vi "MecaOdometry_Execute.vi"(6 "Initial Pose":T1={"TRANSLATION"={"X"=0.0, "Y"=0.0}, "ROTATION"={"VALUE"=0.0, "COS"=1.0, "SIN"=0.0}} {"ROTATION"."SIN" format="%13.4f"; "ROTATION"."COS" format="%13.4f"; "ROTATION"."VALUE" format="%13.4f"; "TRANSLATION"."Y" format="%14.3f"; "TRANSLATION"."X" format="%14.3f"}, 8 "Init":bool, 9 "Rotation":T3={"VALUE"=0.0, "COS"=1.0, "SIN"=0.0} {"SIN" format="%13.4f"; "COS" format="%13.4f"; "VALUE" format="%13.4f"}, 10 "Meca Module Positions":T4 {"RearRight" format="%19.3f"; "RearLeft" format="%19.3f"; "FrontRight" format="%19.3f"; "FrontLeft" format="%19.3f"}, 11 "MECA_DRIVE_KINEMATICS":T5={"FrontLeft"={"X"=0.0, "Y"=0.0}, "FrontRight"={"X"=0.0, "Y"=0.0}, "RearLeft"={"X"=0.0, "Y"=0.0}, "RearRight"={"X"=0.0, "Y"=0.0}, "InverseKinematics"=[[0.0, 1.0, -1.0, 0.0], [0.0, 1.0, 1.0, 0.0], [0.0, 1.0, 1.0, 0.0], [0.0, 1.0, -1.0, 0.0]], "ForwardKinematics"=[[0.0, 1.0, -1.0, 0.0], [0.0, 1.0, 1.0, 0.0], [0.0, 1.0, 1.0, 0.0], [0.0, 1.0, -1.0, 0.0]], "PrevCoR"={"X"=0.0, "Y"=0.0}} {"PrevCoR"."Y" format="%14.3f"; "PrevCoR"."X" format="%14.3f"; "RearRight"."Y" format="%14.3f"; "RearRight"."X" format="%14.3f"; "RearLeft"."Y" format="%14.3f"; "RearLeft"."X" format="%14.3f"; "FrontRight"."Y" format="%14.3f"; "FrontRight"."X" format="%14.3f"; "FrontLeft"."Y" format="%14.3f"; "FrontLeft"."X" format="%14.3f"}) -> (3 "Current Pose":T1={"TRANSLATION"={"X"=0.0, "Y"=0.0}, "ROTATION"={"VALUE"=0.0, "COS"=1.0, "SIN"=0.0}} {"ROTATION"."SIN" format="%13.4f"; "ROTATION"."COS" format="%13.4f"; "ROTATION"."VALUE" format="%13.4f"; "TRANSLATION"."Y" format="%14.3f"; "TRANSLATION"."X" format="%14.3f"}, 4 "MECA_DRIVE_ODOMETRY":T7={"POSE"={"TRANSLATION"={"X"=0.0, "Y"=0.0}, "ROTATION"={"VALUE"=0.0, "COS"=1.0, "SIN"=0.0}}, "GyroOffset"={"VALUE"=0.0, "COS"=1.0, "SIN"=0.0}, "PreviousAngle"={"VALUE"=0.0, "COS"=1.0, "SIN"=0.0}, "Kinematics"={"FrontLeft"={"X"=0.0, "Y"=0.0}, "FrontRight"={"X"=0.0, "Y"=0.0}, "RearLeft"={"X"=0.0, "Y"=0.0}, "RearRight"={"X"=0.0, "Y"=0.0}, "InverseKinematics"=[[0.0, 1.0, -1.0, 0.0], [0.0, 1.0, 1.0, 0.0], [0.0, 1.0, 1.0, 0.0], [0.0, 1.0, -1.0, 0.0]], "ForwardKinematics"=[[0.0, 1.0, -1.0, 0.0], [0.0, 1.0, 1.0, 0.0], [0.0, 1.0, 1.0, 0.0], [0.0, 1.0, -1.0, 0.0]], "PrevCoR"={"X"=0.0, "Y"=0.0}}, "PreviousWheelPositions"={"FrontLeft"=0.0, "FrontRight"=0.0, "RearLeft"=0.0, "RearRight"=0.0, "P"=FALSE}} {"PreviousWheelPositions"."RearRight" format="%19.3f"; "PreviousWheelPositions"."RearLeft" format="%19.3f"; "PreviousWheelPositions"."FrontRight" format="%19.3f"; "PreviousWheelPositions"."FrontLeft" format="%19.3f"; "Kinematics"."PrevCoR"."Y" format="%14.3f"; "Kinematics"."PrevCoR"."X" format="%14.3f"; "Kinematics"."RearRight"."Y" format="%14.3f"; "Kinematics"."RearRight"."X" format="%14.3f"; "Kinematics"."RearLeft"."Y" format="%14.3f"; "Kinematics"."RearLeft"."X" format="%14.3f"; "Kinematics"."FrontRight"."Y" format="%14.3f"; "Kinematics"."FrontRight"."X" format="%14.3f"; "Kinematics"."FrontLeft"."Y" format="%14.3f"; "Kinematics"."FrontLeft"."X" format="%14.3f"; "PreviousAngle"."SIN" format="%13.4f"; "PreviousAngle"."COS" format="%13.4f"; "PreviousAngle"."VALUE" format="%13.4f"; "GyroOffset"."SIN" format="%13.4f"; "GyroOffset"."COS" format="%13.4f"; "GyroOffset"."VALUE" format="%13.4f"; "POSE"."ROTATION"."SIN" format="%13.4f"; "POSE"."ROTATION"."COS" format="%13.4f"; "POSE"."ROTATION"."VALUE" format="%13.4f"; "POSE"."TRANSLATION"."Y" format="%14.3f"; "POSE"."TRANSLATION"."X" format="%14.3f"})   [LabVIEW 2019, in "Trajectory_Library.lvlib"]
doc: "SIngle call LabVIEW function to execute Mecanum Drive Odometry to calculate a relative or absolute POSE.\n \nInputs:\n - Mecanum_Drive_Kinematics -- cluster -- mecanum drive kinematics\n - Mecanum Wheel Positions -- array of cluster -- current wheel positions (distances).\n - Gyro Value -- rotation2d -- current gyro reading.\n - Init -- boolean -- Reset position to the value of Initial Pose. Odometry is calculated from this position.\n - Initial Pose -- Pose2d -- Pose to use when Init is TRUE. (Optional. Default: 0,0,0 )\n\nReturns\n - Current Pose -- Pose2d -- Current position calculated by Mecanum Odometry\n - Mecanum_Drive_Odometry -- cluster -- current value of the mecanum drive odometry cluster."
uses:
  TypeDef/POSE2D.ctl
  TypeDef/TRANSLATION2D.ctl
  TypeDef/ROTATION2D.ctl
  <vilib>/Analysis/Matrix/Datatypes/RealMatrix.ctl
  Pose2d_getRotation.vi
  Rotation2d_Minus.vi
  Rotation2d_UnaryMinus.vi
  Rotation2d_RotateBy.vi
  Rotation2d_CreateAngle.vi
  Rotation2d_CreateXY.vi
  Util_CalcDist.vi
  Trajectory_Library.lvlib
  <vilib>/Analysis/Matrix/NI_Matrix.lvlib
  TypeDef/MECA_DRIVE_KINEMATICS.ctl
  TypeDef/MECA_WHEEL_POSITIONS.ctl
  TypeDef/MECA_DRIVE_ODOMETRY.ctl
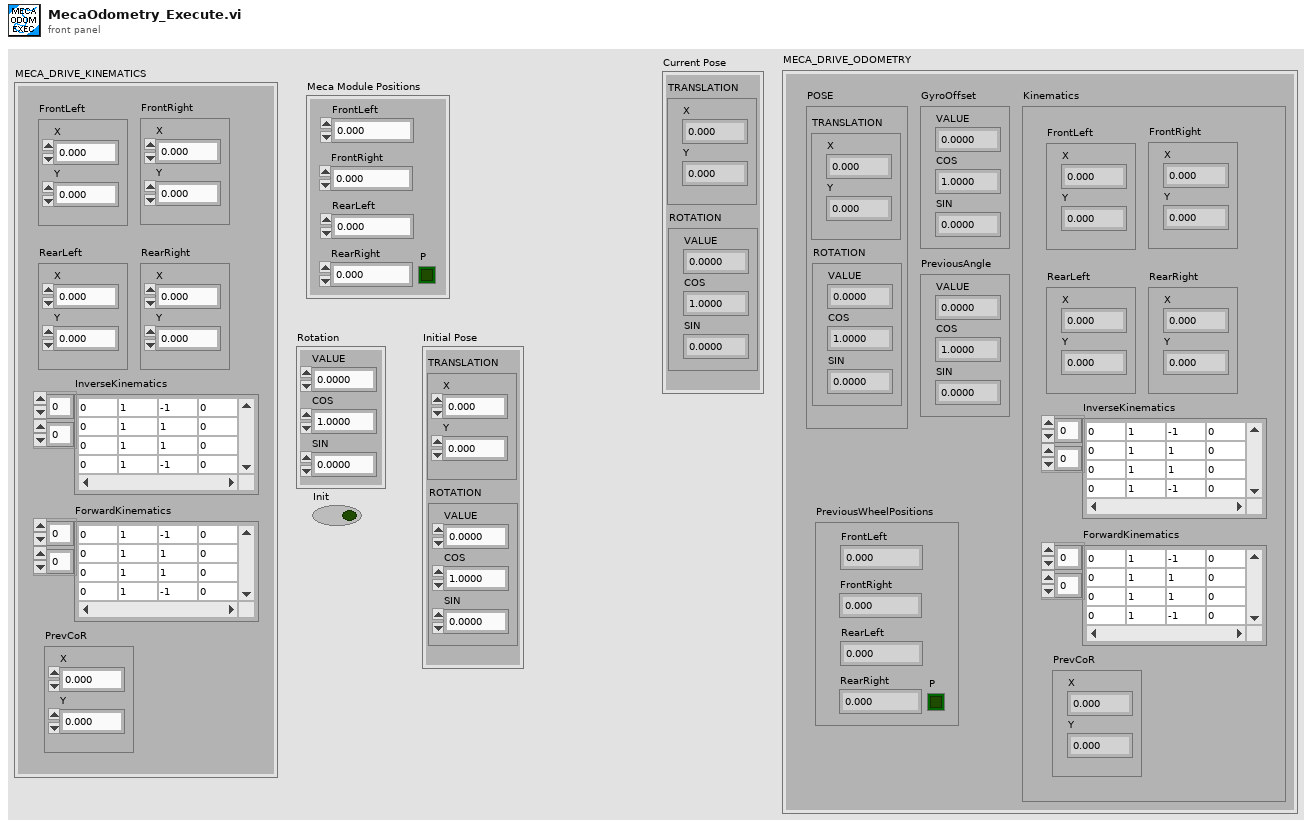
[diagram p1: front panel]
types:
  T1 = typedef "Trajectory_Library.lvlib/POSE2D.ctl" = cluster{"TRANSLATION":T2, "ROTATION":T3}
  T2 = typedef "Trajectory_Library.lvlib/TRANSLATION2D.ctl" = cluster{"X":dbl, "Y":dbl}
  T3 = typedef "Trajectory_Library.lvlib/ROTATION2D.ctl" = cluster{"VALUE":dbl, "COS":dbl, "SIN":dbl}
  T4 = typedef "Trajectory_Library.lvlib/MECA_WHEEL_POSITIONS.ctl" = cluster{"FrontLeft":dbl, "FrontRight":dbl, "RearLeft":dbl, "RearRight":dbl, "P":bool}
  T5 = typedef "Trajectory_Library.lvlib/MECA_DRIVE_KINEMATICS.ctl" = cluster{"FrontLeft":T2, "FrontRight":T2, "RearLeft":T2, "RearRight":T2, "InverseKinematics":T6, "ForwardKinematics":T6, "PrevCoR":T2}
  T6 = typedef "NI_Matrix.lvlib/RealMatrix.ctl" = dbl[][]
  T7 = typedef "Trajectory_Library.lvlib/MECA_DRIVE_ODOMETRY.ctl" = cluster{"POSE":T1, "GyroOffset":T3, "PreviousAngle":T3, "Kinematics":T5, "PreviousWheelPositions":T4}
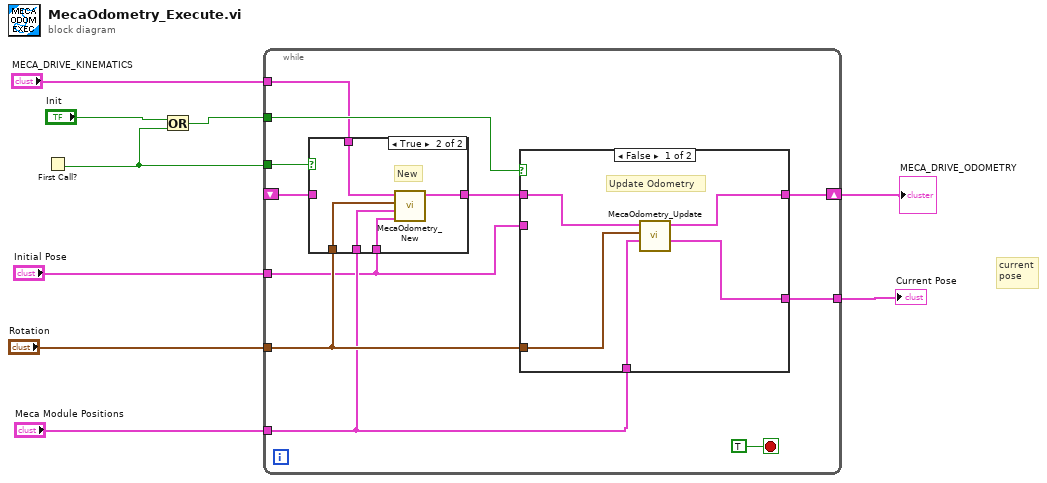
[diagram p0: block diagram]
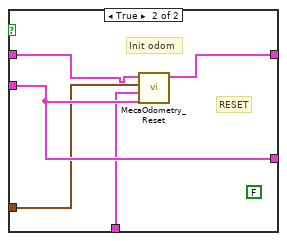
[diagram p3: hidden frame]
diagram:
  # "current\npose"
  n1 = First Call?() -> (First Call?: T/F=w7:bool)
  n2 = Or(x="Init", y=w7) -> (x .or. y?=w8:bool)
  n3 = while {
    tunnel: "Meca Module Positions" -> [w14]
    tunnel: "Rotation" -> [w15]
    tunnel: "MECA_DRIVE_KINEMATICS" -> [w10]
    tunnel: [w17] -> w5
    tunnel: w8 -> [w20]
    shift-right: [w18] -> w6
    shift-left: _ -> [w11]
    tunnel: "Initial Pose" -> [w13]
    tunnel: w7 -> [w16]
    stop <- TRUE stop-if-true
    n4 = case shown="True" w16 {
      tunnel: w15 -> [_ w25]
      tunnel: w14 -> [_ w24]
      tunnel: w13 -> [_ w23]
      tunnel: [w21 w26] -> w12
      tunnel: w11 -> [w21 _]
      tunnel: w10 -> [_ w22]
      frame False {
      }
      frame True {
        # "New"
        n5 = call "MecaOdometry_New.vi"("Initial Pose2d"=w23, "wheelPositions"=w24, "GyroOffset"=w25, "Mecanum Kinematics"=w22) -> ("MECA_DRIVE_ODOMETRY"=w26:T7)  [unwired: 7 in]
      }
    }
    n6 = case shown="False" w20 {
      tunnel: w12 -> [w27 w35]
      tunnel: w15 -> [w28 w33]
      tunnel: w14 -> [w29 w32]
      tunnel: [w30 w36] -> w18
      tunnel: [w31 w34] -> w17
      tunnel: w13 -> [_ w34]
      frame False {
        # "Update Odometry"
        n7 = call "MecaOdometry_Update.vi"("WheelPosition"=w29, "GyroAngle"=w28, "in MECA_DRIVE_ODOMETRY"=w27) -> ("POSE"=w31:T1, "out MECA_DRIVE_ODOMETRY"=w30:T7)  [unwired: 7 in]
      }
      frame True {
        (unwired) FALSE ("Error")
        # "RESET"
        # "Init odom"
        n8 = call "MecaOdometry_Reset.vi"("POSE"=w34, "WheelPositions"=w32, "GyroOffset"=w33, "in MECA_DRIVE_ODOMETRY"=w35) -> ("out MECA_DRIVE_ODOMETRY"=w36:T7)  [unwired: 7 in]
      }
    }
  }
  "MECA_DRIVE_ODOMETRY" <- w6
  "Current Pose" <- w5
